vi "get Request Channel.vi"(8 "error in (no error)":errorcluster, 11 "Actor in":refnum<class "Actor.lvclass">) -> (0 "error out":errorcluster, 2 "Request Channel":refnum<class "Messenger.lvclass">, 3 "Actor out":refnum<class "Actor.lvclass">)   [LabVIEW 2015, in "Actor.lvclass"]
uses:
  Actor.lvclass
  Messaging/Messenger/Messenger.lvclass
  Actor.lvclass/Actor.ctl
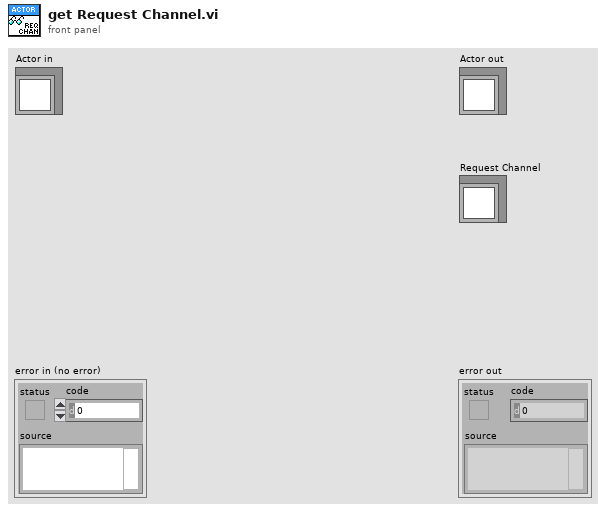
[diagram p1: front panel]
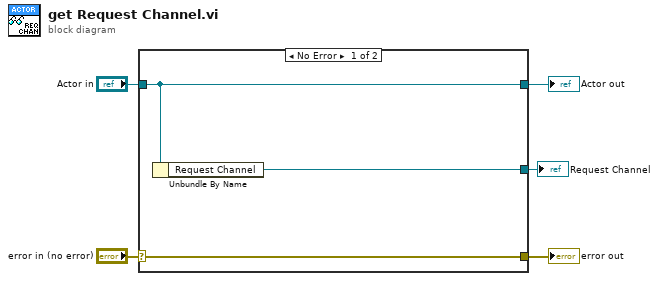
[diagram p0: block diagram]
diagram:
  n1 = case shown="No Error" "error in (no error)" {
    selector: "error in (no error)" -> [w8 w9]
    tunnel: [w8 w9] -> w4
    tunnel: [w7 w10] -> w2
    tunnel: "Actor in" -> [w7 w10]
    tunnel: [w6 _] -> w1
    frame No Error {
      n2 = Unbundle By Name(w7) -> ("Request Channel"=w6:refnum<class "Messenger.lvclass">)
    }
    frame Error {
    }
  }
  "error out" <- w4
  "Actor out" <- w2
  "Request Channel" <- w1
